vi "external cmd - main.vi"(7 "error":string, 13 "option":T2(ring)) -> (4 "address":u8, 6 "content":string, 8 "is true":bool, 10 "cmd available":bool)   [LabVIEW 2010]
uses:
  <vilib>/Utility/error.llb/whitespace.ctl
panel:
  out "line of last command":i32
  out "last command (raw)":string
  out "commands available":T1
  out "current file path":path
  out "freeze":bool
  out "commands pending":bool
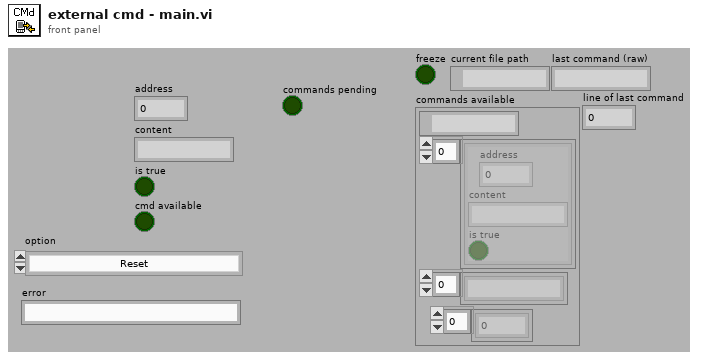
[diagram p1: front panel]
types:
  T1 = cluster{path, cluster{"address":u8, "content":string, "is true":bool}[], string[], i32[]}
  T2 = enum16{"Reset", "Get command", "Open files", "Freeze", "Unfreeze", "Save error"}
  T3 = cluster{path, cluster{"address":u8, "content":string, "is true":bool, i32, string}[]}
  T4 = typedef "whitespace.ctl" = u16
  T5 = cluster{"address":u8, "content":string, "is true":bool, i32, string}[]
  T6 = cluster{"address":u8, "content":string, "is true":bool, i32, string}
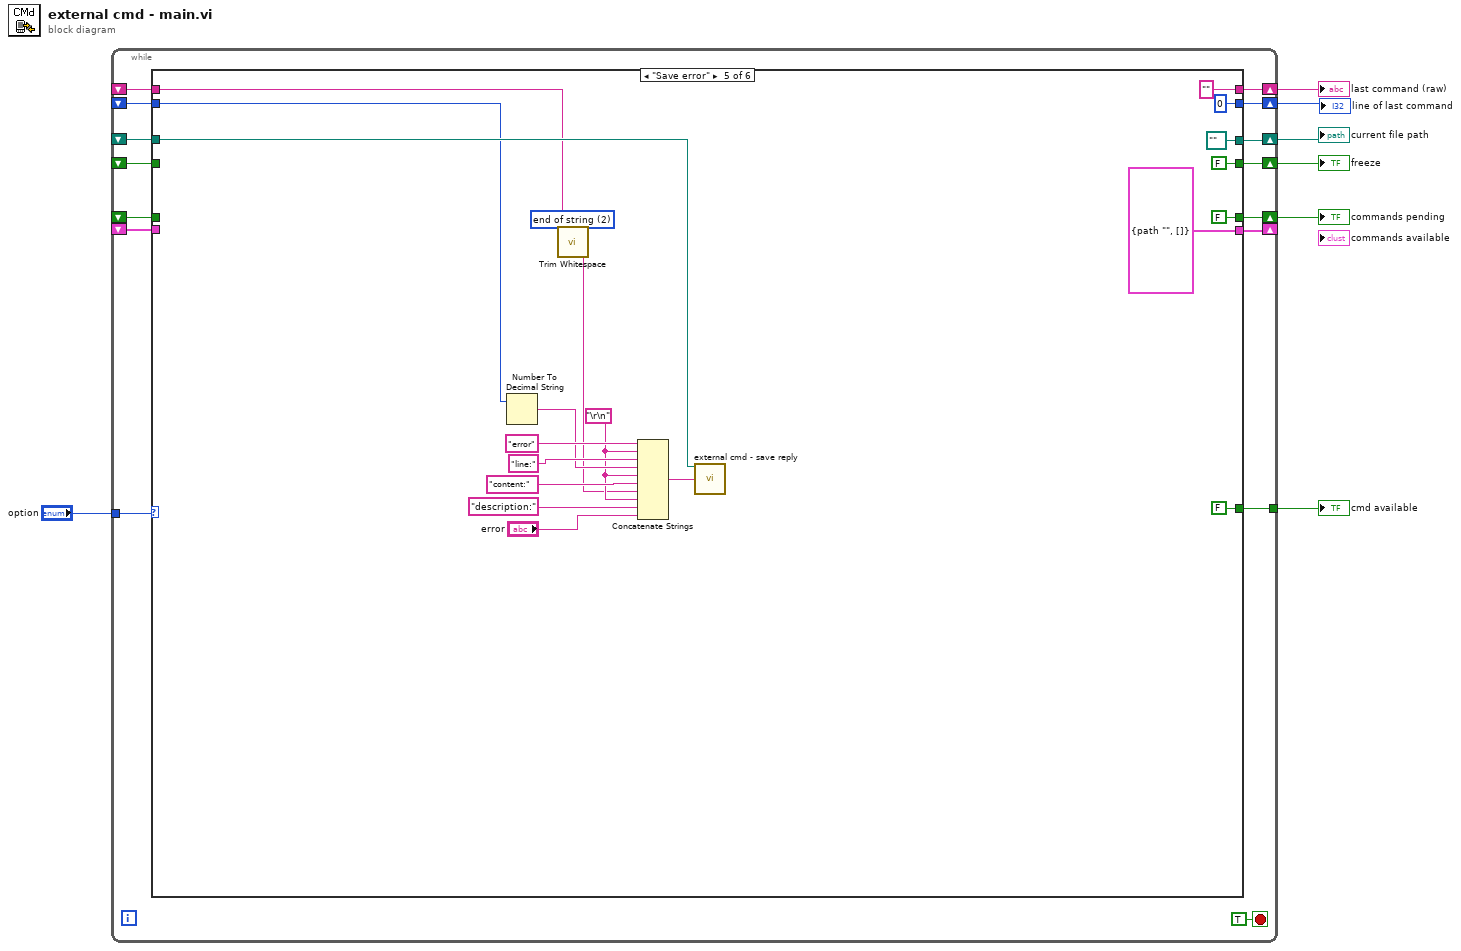
[diagram p0: block diagram]
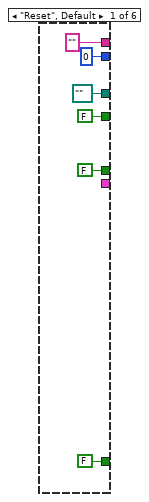
[diagram p2: hidden frame]
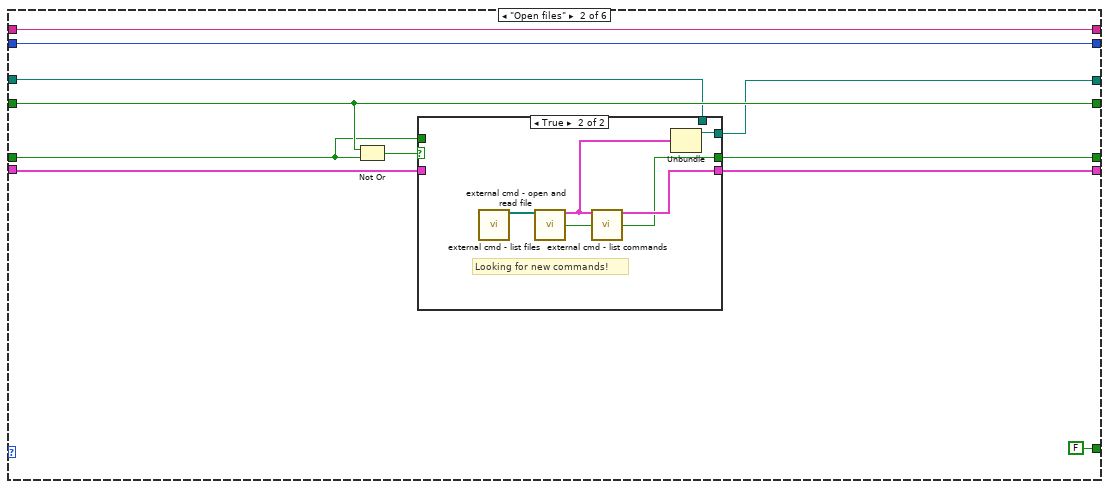
[diagram p3: hidden frame]
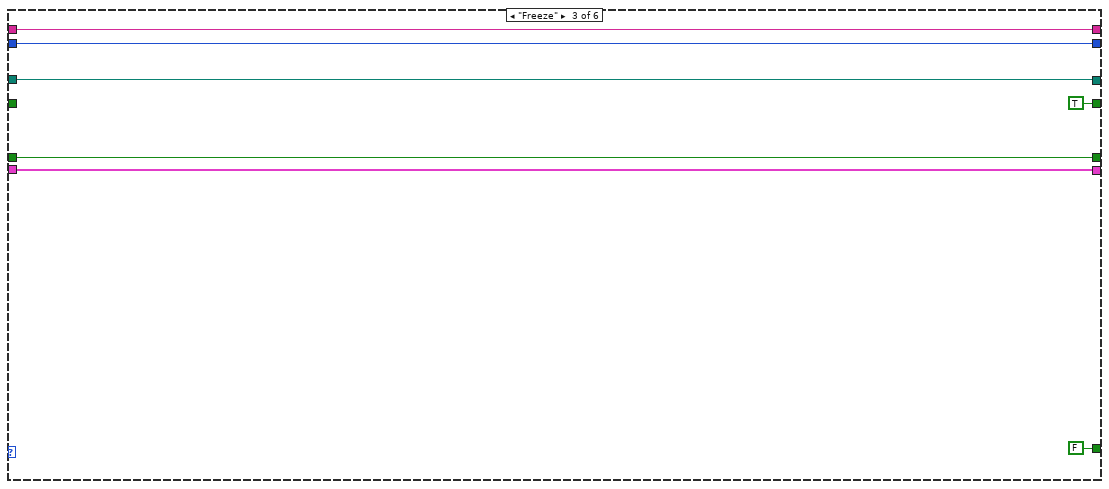
[diagram p5: hidden frame]
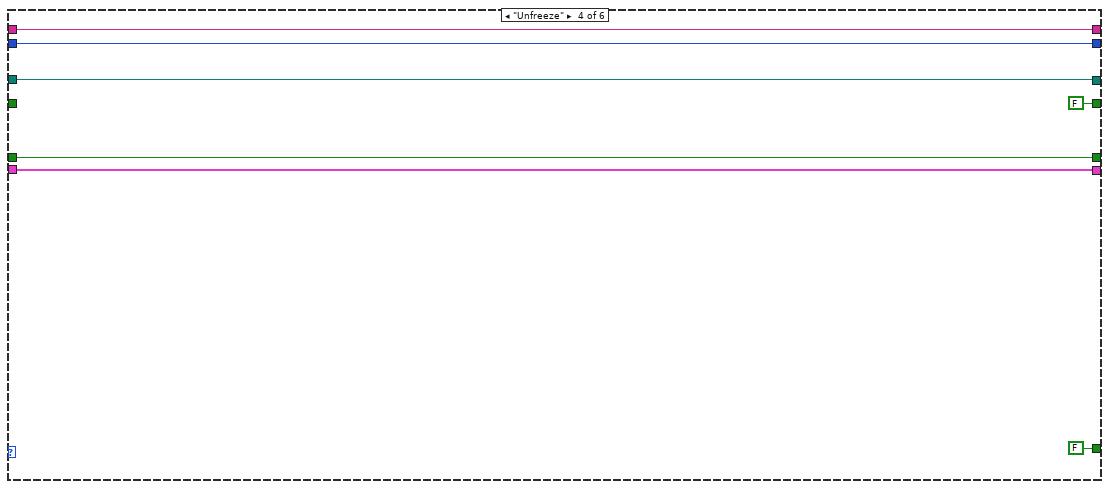
[diagram p6: hidden frame]
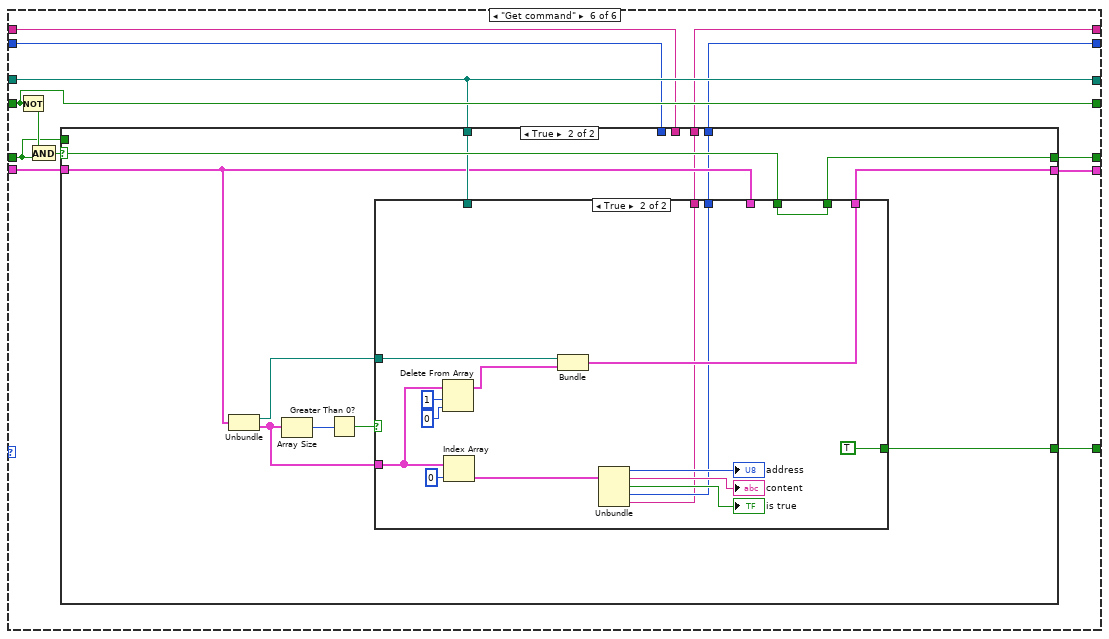
[diagram p7: hidden frame]
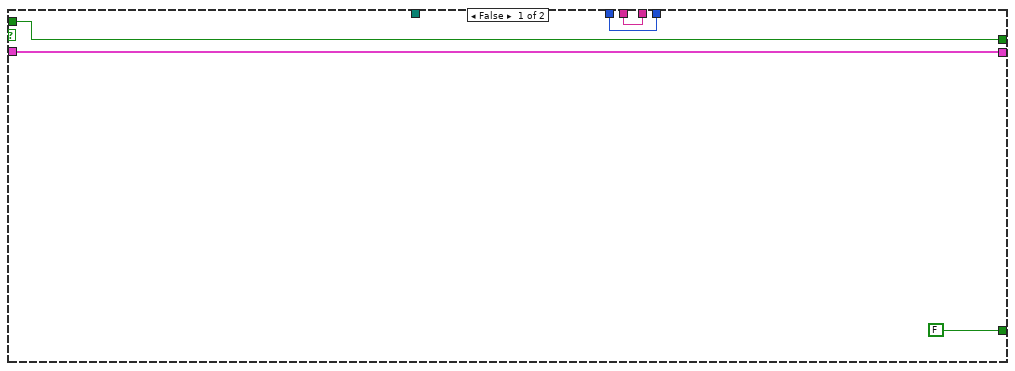
[diagram p8: hidden frame]
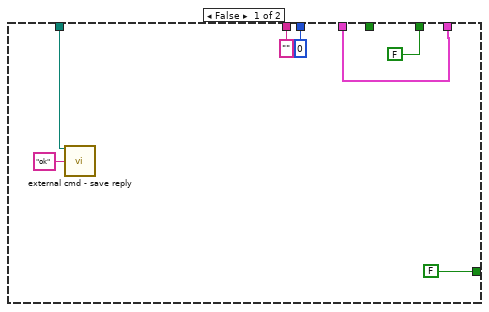
[diagram p9: hidden frame]
diagram:
  n1 = while {
    shift-right: [w20] -> w5
    shift-left: _ -> [w21]
    shift-right: [w19] -> _
    shift-left: _ -> [w18]
    tunnel: [w17] -> w7
    tunnel: "option" -> [w16]
    shift-right: [w15] -> w4
    shift-left: _ -> [w14]
    shift-right: [w13] -> w3
    shift-left: _ -> [w12]
    shift-right: [w10] -> w1
    shift-left: _ -> [w9]
    shift-right: [w11] -> w2
    shift-left: _ -> [w8]
    stop <- TRUE stop-if-true
    n2 = case shown="\"Save error\"" w16 {
      tunnel: w21 -> [_ w33 w54 w61 _ w88]
      tunnel: [FALSE ("has commands") w38 w54 w61 FALSE ("has commands") w92] -> w20
      tunnel: [_ w39 w53 w60 T3 {path "", []} ("commands") w95] -> w19
      tunnel: w18 -> [_ w36 w53 w60 _ w94]
      tunnel: [FALSE ("is true 2") FALSE ("is true 2") FALSE ("is true 2") FALSE ("is true 2") FALSE ("is true 2") w93] -> w17
      tunnel: [FALSE ("has commands") w34 TRUE ("has commands") FALSE ("has commands") FALSE ("has commands") w89] -> w15
      tunnel: w14 -> [_ w34 _ _ _ w89]
      tunnel: [path "" w32 w51 w58 path "" w87] -> w13
      tunnel: w12 -> [_ w31 w51 w58 w81 w87]
      tunnel: ["" w30 w49 w56 "" w86] -> w11
      tunnel: [0 w29 w50 w57 0 w85] -> w10
      tunnel: w9 -> [_ w29 w50 w57 w74 w83]
      tunnel: w8 -> [_ w30 w49 w56 w71 w84]
      frame "Reset", Default {
      }
      frame "Open files" {
        n3 = Not Or(1:w33, 2:w34) -> (0:w35:bool)
        n4 = case shown="True" w35 {
          tunnel: [w42 w46] -> w39
          tunnel: [w41 w45] -> w38
          tunnel: w36 -> [w42 _]
          tunnel: w33 -> [w41 _]
          tunnel: [w40 w44] -> w32
          tunnel: w31 -> [w40 _]
          frame False {
          }
          frame True {
            # "Looking for new commands!"
            n5 = call "external cmd - list files.vi"() -> ("files array"=w47:path[])  [unwired: 15 in]
            n6 = call "external cmd - open and read file.vi"("files array"=w47) -> ("commands"=w43:cluster{path, string[], i32[]}, "file has commands"=w48:bool)  [unwired: 13 in]
            n7 = call "external cmd - list commands.vi"("commands"=w43, "file has commands"=w48) -> ("commands"=w46:T3, "has commands"=w45:bool)  [unwired: 12 in]
            n8 = Unbundle(w43) -> (w44:path)  [unwired: 2 out]
          }
        }
      }
      frame "Freeze" {
      }
      frame "Unfreeze" {
      }
      frame "Save error" {
        w64 = T4 2 items=["both", "start of string", "end of string"] ("location (both)")
        w70 = "\r\n"
        n9 = Number To Decimal String(number=w74) -> (decimal integer string=w73:string)  [unwired: 1 in]
        n10 = call <vilib>:"Trim Whitespace.vi"("string"=w71, "location (both)"=w64) -> ("trimmed string"=w65:string)
        n11 = Concatenate Strings("error" ("string"), w70, "line:" ("string"), w73, w70, "content:" ("string"), w65, w70, "description:" ("string"), "error") -> (w67:string)
        n12 = call "external cmd - save reply.vi"("Path"=w81, "reply content"=w67) -> ()  [unwired: 14 in]
      }
      frame "Get command" {
        n13 = Not(x=w89) -> (.not. x?=w90:bool)
        n14 = And(x=w90, y=w88) -> (x .and. y?=w91:bool)
        n15 = case shown="True" w91 {
          selector: w91 -> [_ w108]
          tunnel: [w98 w109] -> w92
          tunnel: [w99 w106] -> w95
          tunnel: w94 -> [w99 w103]
          tunnel: [FALSE ("is true 2") w105] -> w93
          tunnel: w88 -> [w98 _]
          tunnel: w87 -> [_ w104]
          tunnel: [w97 w102] -> w86
          tunnel: [w96 w101] -> w85
          tunnel: w84 -> [w97 _]
          tunnel: w83 -> [w96 _]
          frame False {
          }
          frame True {
            n16 = Unbundle(w103) -> (w107:path, w110:T5)
            n17 = Array Size(array=w110) -> (size(s)=w112:i32)
            n18 = Greater Than 0?(x=w112) -> (x > 0?=w111:bool)
            n19 = case shown="True" w111 {
              tunnel: w110 -> [_ w128]
              tunnel: [FALSE ("has commands") w129] -> w109
              tunnel: w108 -> [_ w129]
              tunnel: w107 -> [_ w125]
              tunnel: [w118 w122] -> w106
              tunnel: w103 -> [w118 _]
              tunnel: [FALSE ("is true 2") TRUE ("is true 2")] -> w105
              tunnel: w104 -> [w115 _]
              tunnel: ["" w120] -> w102
              tunnel: [0 w121] -> w101
              frame False {
                n20 = call "external cmd - save reply.vi"("Path"=w115, "reply content"="ok") -> ()  [unwired: 14 in]
              }
              frame True {
                n21 = Delete From Array(array=w128, length=1, index=0) -> (array with subset deleted=w124:T5)  [unwired: 1 out]
                n22 = Index Array(array=w128, index=0) -> (element=w133:T6)
                n23 = Bundle(w125, w124) -> (w122:T3)  [unwired: 1 in]
                n24 = Unbundle(w133) -> ("address"=→"address":u8, "content"=→"content":string, "is true"=→"is true":bool, w121:i32, w120:string)
              }
            }
          }
        }
      }
    }
  }
  "cmd available" <- w7
  "commands pending" <- w5
  "freeze" <- w4
  "current file path" <- w3
  "last command (raw)" <- w2
  "line of last command" <- w1
